vi "Traccia_Vin_Vout_2015diff.vi"() -> ()   [LabVIEW 2014]
doc: "Traccia_Vin_Vout\nUtilizza Vin_Vout e traccia una curva Vout vs Vin\n9/2011, 9/2015 vers. LV2014 \nFM & ADL"
uses:
  <vilib>/Utility/file.llb/Write To Spreadsheet File (DBL).vi
panel:
  in  "Fondo Scala AI1":dbl(ring)=10.0 items=["10"=10.0, "5"=5.0, "0.5"=0.5, "0.05"=0.05]
  in  "Scala Asse Y":enum8{"Lineare", "Logaritmica"}(ring)
  in  "R (kOhm)":dbl=2.2 min=-10.0 max=10.0 step=0.1 format="%_4g"
  in  "Fondo Scala AI0":dbl(ring)=10.0 items=["10"=10.0, "5"=5.0, "0.5"=0.5, "0.05"=0.05]
  in  "SALVA I DATI SU FILE":bool=TRUE caption="ON\nOFF"
  out "N. misura":i16
  out "Corrente in funzione della tensione ai capi":cluster{dbl[], dbl[]}(graph)
  out "Vin (V)":dbl format="%_4g"
  out "V_L (V)":dbl format="%_4f"
  in  "Numero misure":i16=10 min=0 max=1000 step=1
  in  "Vmax(V)x":dbl=5.0 min=-10.0 max=10.0 step=0.1 format="%_4g"
  in  "Vmin(V)":dbl=-5.0 min=-10.0 max=10.0 step=0.1 format="%_4g"
  # "1) Scegliere il fondo scala dei due ingressi analogici"
  # "Collegare il CB 22 (analog output) e il CB68 (AI0) all'ingresso Vin\n  \nCollegare i CB33 e CB34 all'uscita Vout . \n\nLa terra del circuito (CB29) DEVE essere in comune alla terra della scheda."
  # "2) Selezionare il valore minimo e massimo della tensione di ingresso ed il numero di valori (equispaziati  tra gli estremi)"
  # "3) Premere la freccia bianca"
  # "Durante la misura gli indicatori  mostrano i valori di Vin e Vout ed il numero progressivo della misura"
  # "Sul grafico viene mostrata la corrente che scorre nel carico in funzione della tensione ai suoi capi."
  # "NO\nSI"
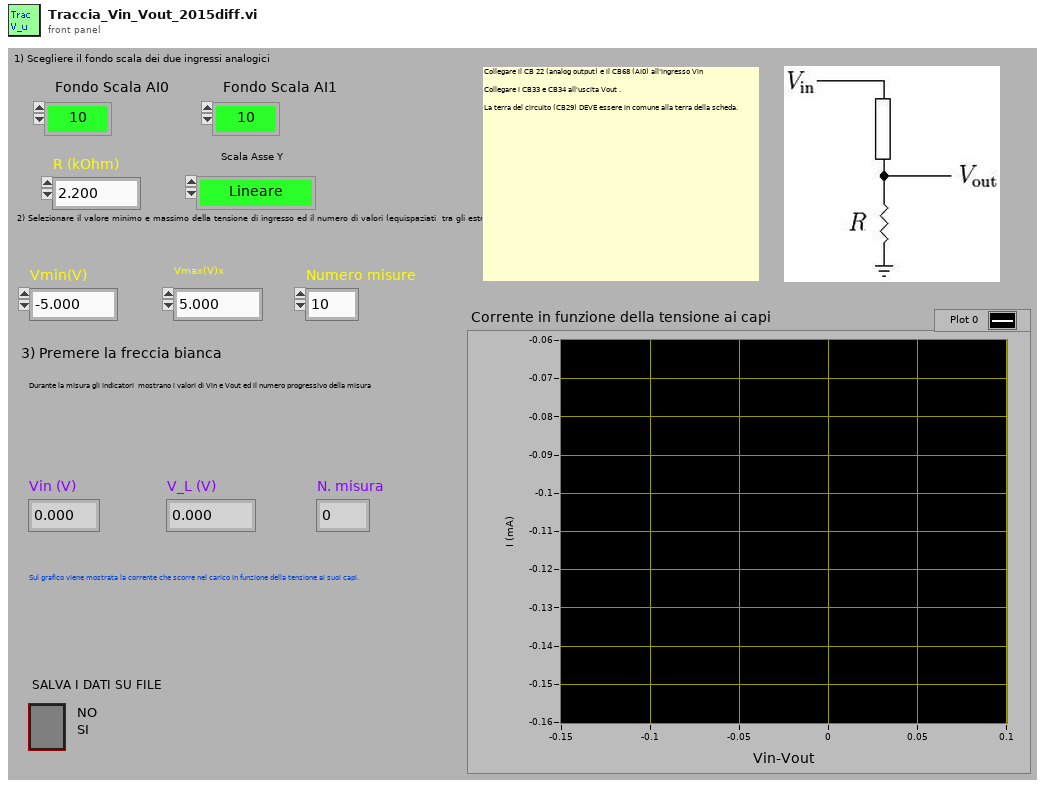
[diagram p1: front panel]
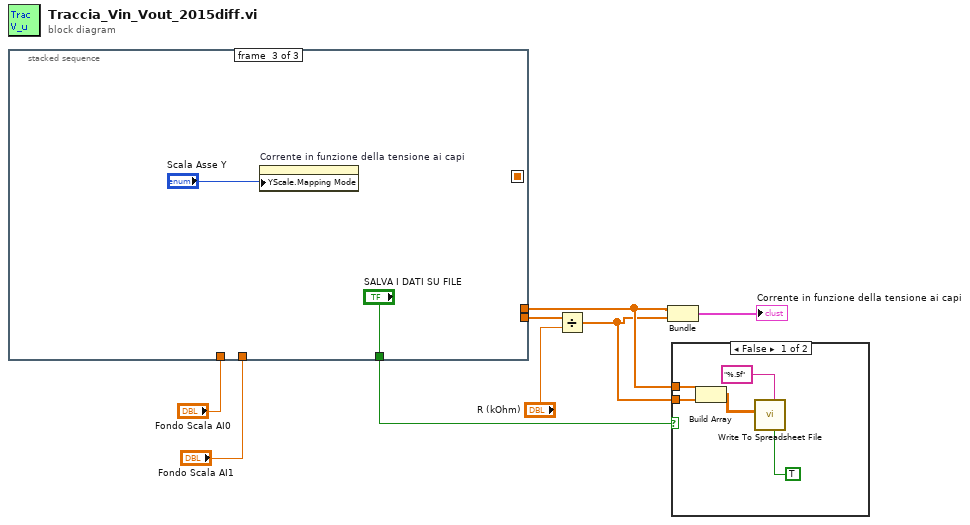
[diagram p0: block diagram]
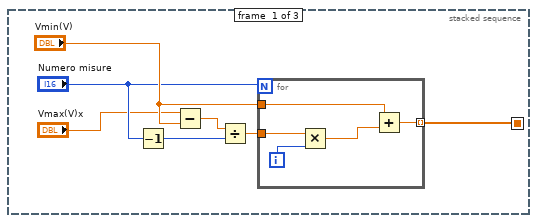
[diagram p3: hidden frame]
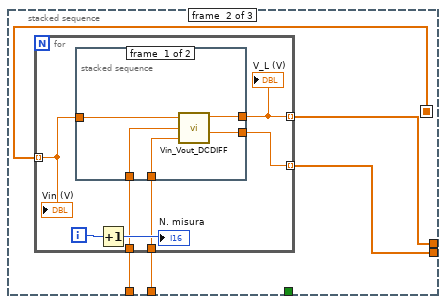
[diagram p4: hidden frame]
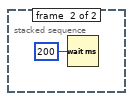
[diagram p5: hidden frame]
diagram:
  n1 = stacked-sequence {
    seq-local: [w11 _ _] -> [_ w24 _]
    tunnel: [_ w21 _] -> w4
    tunnel: [_ w22 _] -> w7
    tunnel: "Fondo Scala AI0" -> [_ w25 _]
    tunnel: "Fondo Scala AI1" -> [_ w23 _]
    tunnel: [_ _ "SALVA I DATI SU FILE"] -> w1
    frame #0 {
      n2 = Decrement(x="Numero misure") -> (x-1=w14:i16)
      n3 = Subtract(x="Vmax(V)x", y="Vmin(V)") -> (x-y=w15:dbl)
      n4 = Divide(x=w15, y=w14) -> (x/y=w13:dbl)
      n5 = for {
        N: "Numero misure" -> [_]
        tunnel: "Vmin(V)" -> [w20]
        tunnel: [w19] -> w11 mode=indexing
        tunnel: w13 -> [w18]
        i -> [w17]
        n6 = Multiply(x=w18, y=w17) -> (x*y=w16:dbl)
        n7 = Add(x=w20, y=w16) -> (x+y=w19:dbl)
      }
    }
    frame #1 {
      n8 = for {
        tunnel: w24 -> [w32] mode=indexing
        tunnel: w25 -> [w29]
        tunnel: w23 -> [w28]
        tunnel: [w26] -> w22 mode=indexing
        tunnel: [w27] -> w21 mode=indexing
        i -> [w31]
        n9 = stacked-sequence {
          tunnel: w32 -> [w36 _]
          tunnel: [w37 _] -> w26
          tunnel: w29 -> [w35 _]
          tunnel: w28 -> [w34 _]
          tunnel: [w33 _] -> w27
          frame #0 {
            n10 = call "Vin_Vout_DCDIFF.vi"("V in volt"=w36, "Fondo Scala AI0 (68-34)"=w35, "Fondo Scala AI1 (33)"=w34) -> ("V0 medio"=w37:dbl, "V1 medio"=w33:dbl)  [unwired: 2 out]
          }
          frame #1 {
            n11 = Wait (ms)(milliseconds to wait=u32 200) -> ()  [unwired: 1 out]
          }
        }
        "V_L (V)" <- w26
        n12 = Increment(x=w31) -> (x+1=→"N. misura":i32)
        "Vin (V)" <- w32
      }
    }
    frame #2 {
      n13 = property on="Corrente in funzione della tensione ai capi" class="XYGraph (strict)"("YScale.Mapping Mode"="Scala Asse Y") -> ()  [unwired: 2 in, 2 out]
    }
  }
  n14 = Divide(x=w4, y="R (kOhm)") -> (x/y=w5:dbl[])
  n15 = Bundle(w7, w5) -> (→"Corrente in funzione della tensione ai capi":cluster{dbl[], dbl[]})  [unwired: 1 in]
  n16 = case shown="False" w1 {
    tunnel: w5 -> [w45 _]
    tunnel: w7 -> [w44 _]
    frame False {
      n17 = Build Array(w44, w45) -> (w43:dbl[][])
      n18 = call-poly <vilib>:"Write To Spreadsheet File.vi"("transpose? (no:F)"=TRUE, "format (%.3f)"="%.5f", "2D data"=w43) -> ()  [unwired: 5 in, 1 out]
    }
    frame True {
    }
  }
